vi "Controller Test Bench (2).vi"() -> ()   [LabVIEW 2022 SP3]
doc: "This example demonstrates how to continuously re-generate analog output data from a buffer in your computer's memory.\n\nRefer to your device documentation for pinouts and hardware capabilities."
uses:
  WhiteNoise.ctl
  <vilib>/Utility/error.llb/DialogType.ctl
  <vilib>/DAQmx/write.llb/DAQmx Write (Analog 1D Wfm NChan NSamp).vi
  <vilib>/DAQmx/read.llb/DAQmx Read (Analog Wfm 1Chan NSamp).vi
  <vilib>/DAQmx/create/channels.llb/DAQmx Create Channel (AO-Voltage-Basic).vi
  <vilib>/DAQmx/configure/timing.llb/DAQmx Timing (Sample Clock).vi
  <vilib>/measure/maspectr.llb/FFT Spectrum (Mag-Phase) for N Chan.vi
  <vilib>/DAQmx/miscellaneous.llb/DAQmx Fill In Error Info.vi
  <vilib>/DAQmx/create/channels.llb/DAQmx Create Channel (AI-Acceleration-Accelerometer).vi
  <vilib>/DAQmx/create/channels.llb/DAQmx Create Channel (AI-Force-IEPE Sensor).vi
  <vilib>/DAQmx/create/channels.llb/DAQmx Create Channel (AI-Sound Pressure-Microphone).vi
  <vilib>/measure/maspectr.llb/FFT Spectrum (Mag-Phase) for 1 Chan.vi
  <resource>/objmgr/daqmx.rc
  <vilib>/measure/NI_MABase.lvlib
  <vilib>/measure/NI_MAPro.lvlib
panel:
  in  "Start Output":bool
  out "Boolean 2":bool
  in  "Master Switch":bool
  in  "Start Control":bool
  in  "Start Input":bool
  in  "Tab Control":T1(tab)
  out "Actual Sample Rate":dbl=1000.0 format="%0.2f"
  in  "Physical Channel(s)":tag="Dev1/ao0"
  in  "Min Voltage":dbl=-3.0
  in  "Max Voltage":dbl=3.5
  in  "Sample Clock Source":tag="OnboardClock"
  in  "Sample Rate":dbl=40000.0
  in  "Stop":bool
  in  "Number of Samples":i32=40000
  out "Waveform Graph":waveform(dbl)[](graph)=[{"t0"=timestamp(0 s since 1904-01-01), "dt"=0.001, "Y"=[]}]
  out "Mag":cluster{"f0":dbl, "df":dbl, "magnitude":dbl[]}[](graph)
  out "Phase":cluster{"f0":dbl, "df":dbl, "phase":dbl[]}[](graph)
  in  "?":enum32{"White Noise", "Harmonic"}(tab)
  in  "Cluster":T3={"Seed"=0.0, "Standard Deviation"=0.2, "Reset"=FALSE, "Iterator"=1.0} {"Standard Deviation" format="%0.2p"}
  in  "Cluster 2":T4={"Iterator"=1.0, "Waveform Type"=0, "Frequency"=10.0, "Amplitude"=0.5} {"Amplitude" format="%0.2p"; "Frequency" format="%0.2p"; "Waveform Type" items=["Sine Wave", "Triangle Wave", "Square Wave", "Sawtooth Wave"]}
  in  "Task Type":T5(tab)
  in  "Min Acceleration":dbl=-100.0
  in  "Max Acceleration":dbl=100.0
  in  "Sensitivity [mV/g]":dbl=95.4
  in  "Physical Channel":tag="Dev1/ai0"
  in  "Sample Clock Source":tag="OnboardClock"
  in  "Sample Rate":dbl=40000.0
  in  "Terminal Configuration":i32(ring)=-1 items=["default"=-1, "RSE"=10083, "NRSE"=10078, "Differential"=10106, "Pseudodifferential"=12529]
  in  "Samples per Loop":i32=40000
  in  "Max Sound Pressure Level (dB)":dbl=120.0
  in  "Sound Pressure Units":i32(ring)=10081 items=["Pascals"=10081, "From Custom Scale"=10065]
  in  "Microphone Sensitivity":dbl=10.0
  in  "Sensitivity 2":dbl=50.0
  in  "Min Force":dbl=-100.0
  in  "Max Force":dbl=100.0
  in  "Sensitivity Units  2":i32(ring)=15891 items=["mVolts/N"=15891, "mVolts/lb"=15892]
  in  "Force Units":i32(ring)=15875 items=["Newtons"=15875, "Pounds"=15876, "From Custom Scale"=10065]
  in  "Window":dbl
  out "Boolean":bool
  in  "Restart Aaveraging":bool
  in  "Stop 2":bool
  out "Waveform Graph 2":waveform(dbl)(graph)
  out "Mag 2":cluster{"f0":dbl, "df":dbl, "magnitude":dbl[]}(graph)
  out "Phase 2":cluster{"f0":dbl, "df":dbl, "phase":dbl[]}(graph)
  in  "Reset Averaging":bool
  # "Channel Settings"
  # "Output"
  # "Timing and\nBuffer Settings"
  # "Waveform Settings"
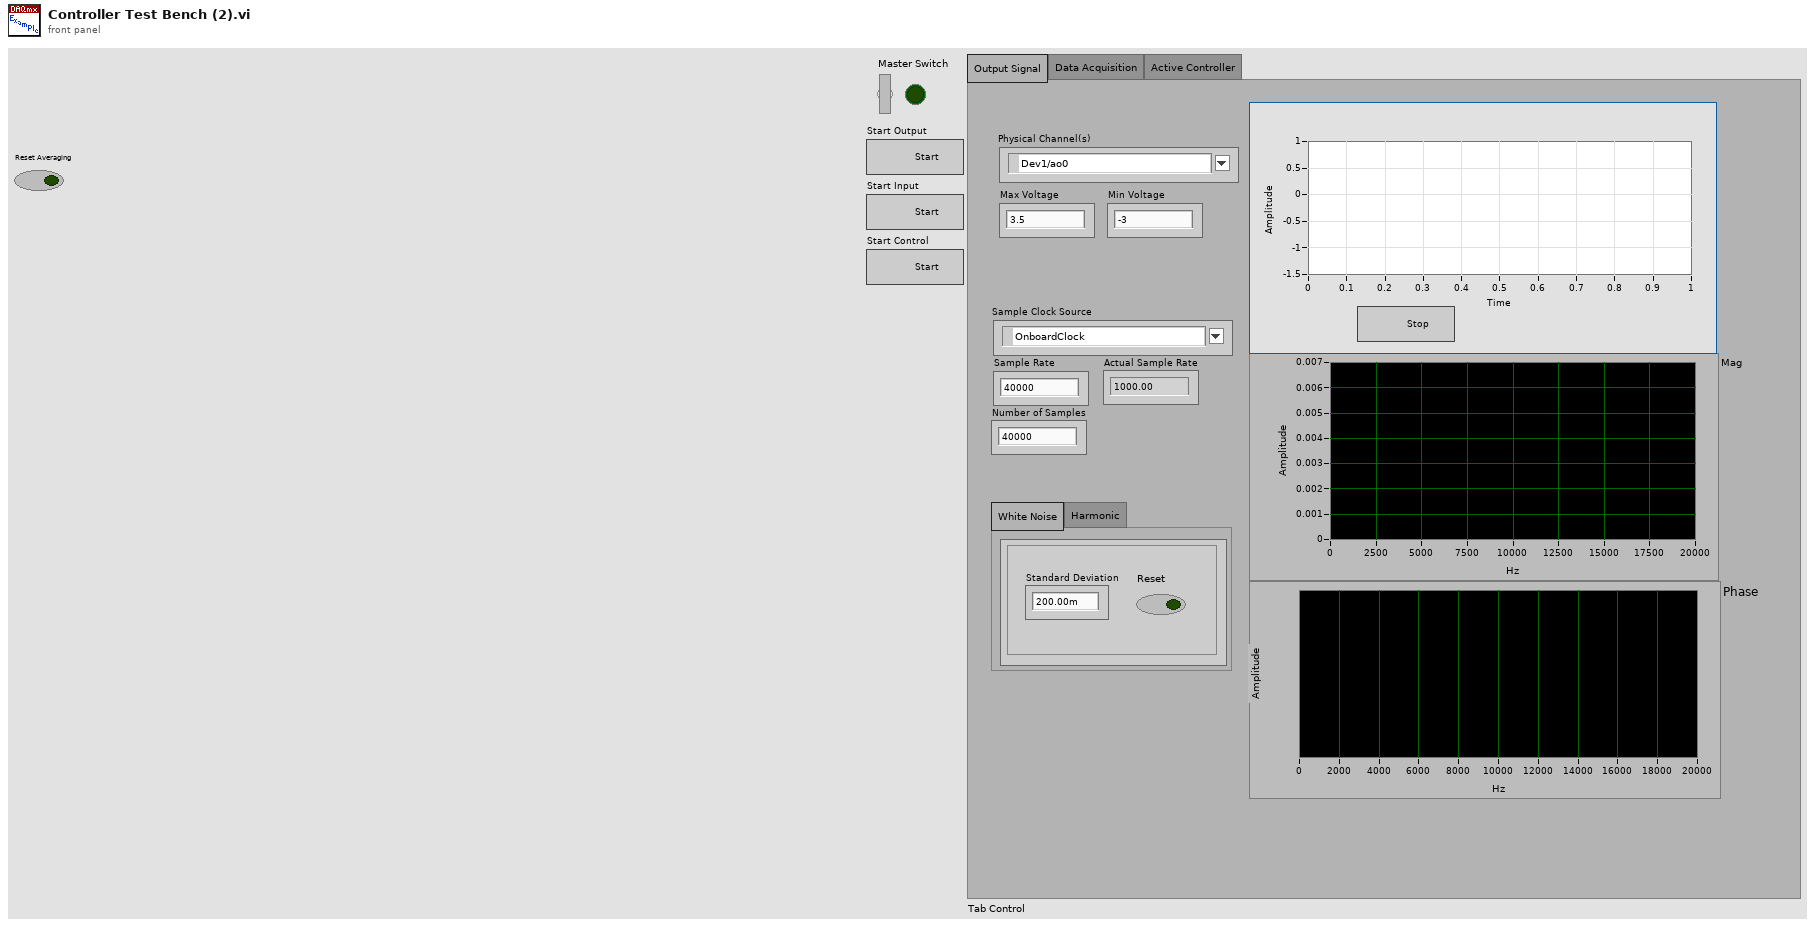
[diagram p1: front panel]
types:
  T1 = enum32{"Output Signal", "Data Acquisition", "Active Controller"}
  T2 = typedef "WhiteNoise.ctl" = dbl
  T3 = cluster{"Seed":T2, "Standard Deviation":dbl, "Reset":bool, "Iterator":dbl}
  T4 = cluster{"Iterator":dbl, "Waveform Type":u16, "Frequency":dbl, "Amplitude":dbl}
  T5 = enum32{"Acceleration", "Sound Pressure", "Force"}
  T6 = typedef "DialogType.ctl" = u16
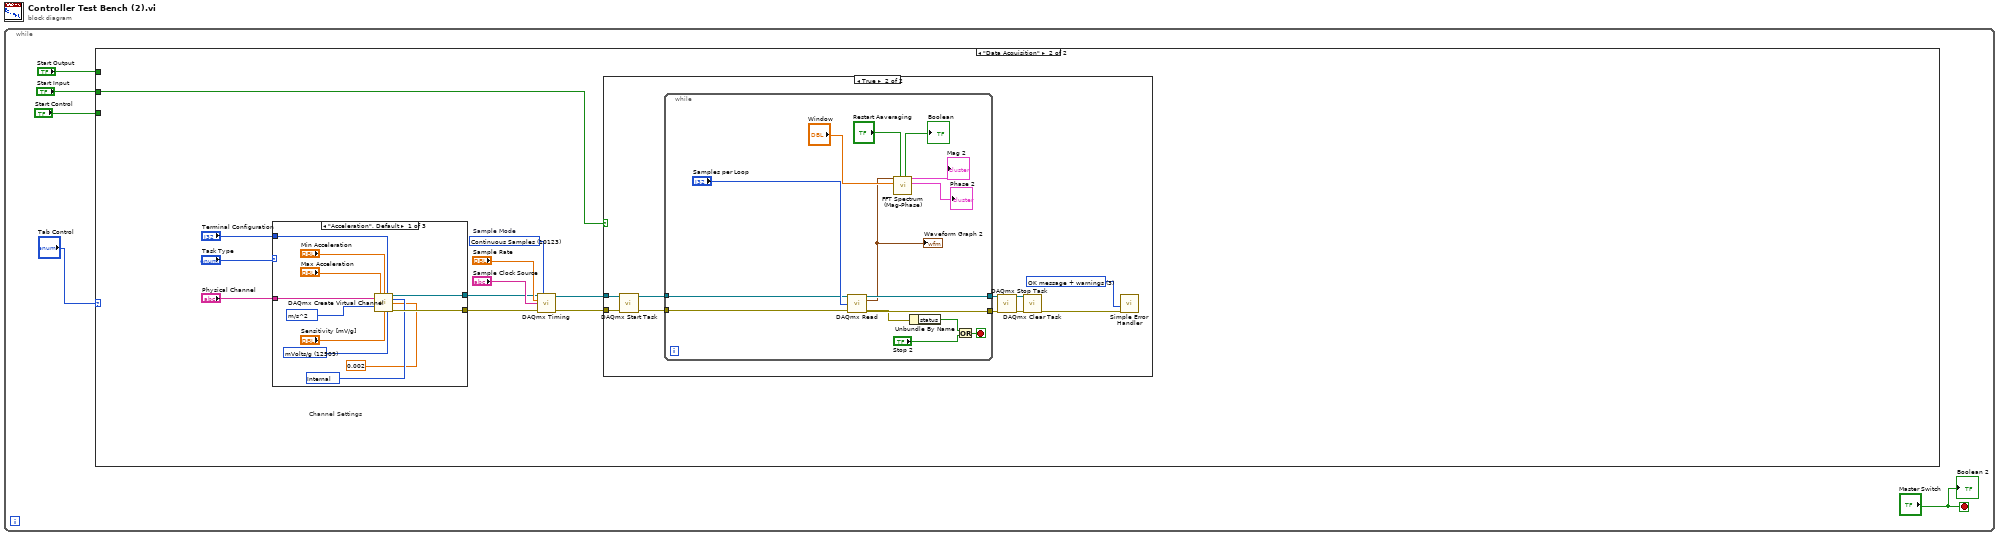
[diagram p0: block diagram]
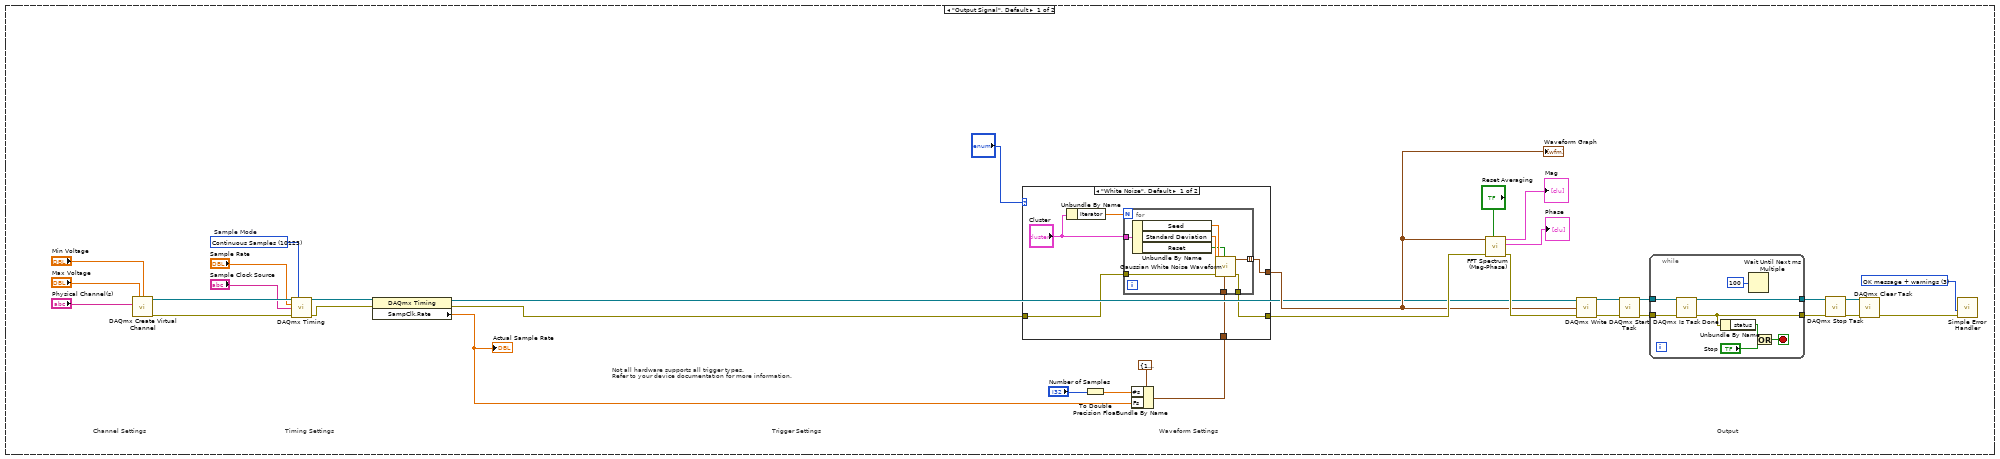
[diagram p2: hidden frame]
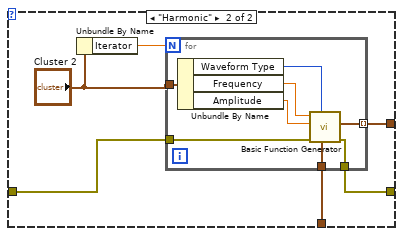
[diagram p3: hidden frame]
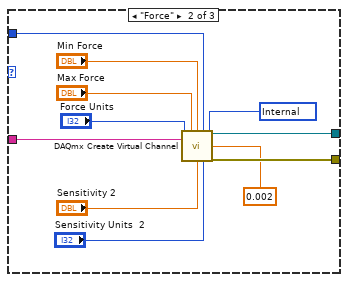
[diagram p5: hidden frame]
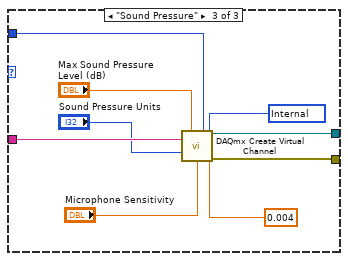
[diagram p6: hidden frame]
diagram:
  n1 = while {
    stop <- "Master Switch" stop-if-true
    n2 = case shown="\"Data Acquisition\"" "Tab Control" {
      tunnel: "Start Output" -> [_ _]
      tunnel: "Start Input" -> [_ w76]
      tunnel: "Start Control" -> [_ _]
      frame "Output Signal", Default {
        w16 = T6 3 items=["no dialog", "OK message", "continue or stop message", "OK message + warnings", "continue/stop + warnings"] ("type of dialog (OK msg:1)")
        w37 = 10123 items=["Finite Samples"=10178, "Continuous Samples"=10123, "Hardware Timed Single Point"=12522]  # Sample Mode
        # "Trigger Settings"
        # "Not all hardware supports all trigger types.\nRefer to your device documentation for more information."
        # "Output"
        # "Waveform Settings"
        # "Timing Settings"
        # "Channel Settings"
        n3 = call-poly <vilib>:"DAQmx Create Virtual Channel.vi"("maximum value"="Max Voltage", "minimum value"="Min Voltage", "physical channels"="Physical Channel(s)") -> ("task out"=w35:refnum<k21>, "error out"=w36:errorcluster)  [unwired: 11 in]
        n4 = call-poly <vilib>:"DAQmx Timing.vi"("task/channels in"=w35, "sample mode"=w37, "rate"="Sample Rate", "source"="Sample Clock Source", "error in"=w36) -> ("task out"=w39:refnum<k21>, "error out"=w38:errorcluster)  [unwired: 9 in]
        n5 = property class="DAQmx Timing"(reference=w39, error in=w38) -> (reference out=w7:refnum<k21>, error out=w6:errorcluster, "SampClk.Rate"=w25:dbl)
        "Actual Sample Rate" <- w25
        n6 = To Double Precision Float(number="Number of Samples") -> (double precision float=w22:dbl)
        n7 = Bundle By Name(cluster=cluster{"Fs":dbl, "#s":dbl} {"Fs"=1000.0, "#s"=1000.0} ("sampling info"), "#s"=w22, "Fs"=w25) -> (w24:cluster{"Fs":dbl, "#s":dbl})
        n8 = case shown="\"White Noise\", Default" "?" {
          tunnel: w24 -> [w45 w57]
          tunnel: w6 -> [w44 w59]
          tunnel: [w43 w56] -> w10
          tunnel: [w40 w58] -> w9
          frame "White Noise", Default {
            n9 = Unbundle By Name("Cluster") -> ("Iterator"=w42:dbl)
            n10 = for {
              N: w42 -> [_]
              tunnel: w44 -> [w53]
              tunnel: w45 -> [w52]
              tunnel: [w51] -> w43
              tunnel: "Cluster" -> [w50]
              tunnel: [w49] -> w40 mode=indexing
              n11 = Unbundle By Name(w50) -> ("Seed"=w48:T2, "Standard Deviation"=w47:dbl, "Reset"=w46:bool)
              n12 = call <vilib>:"Gaussian White Noise Waveform.vi"("sampling info"=w52, "reset signal"=w46, "error in (no error)"=w53, "seed"=w48, "standard deviation"=w47) -> ("error out"=w51:errorcluster, "signal out"=w49:waveform(dbl))  [unwired: 5 in]
            }
          }
          frame "Harmonic" {
            n13 = Unbundle By Name("Cluster 2") -> ("Iterator"=w55:dbl)
            n14 = for {
              N: w55 -> [_]
              tunnel: w59 -> [w67]
              tunnel: w57 -> [w66]
              tunnel: [w65] -> w56
              tunnel: "Cluster 2" -> [w64]
              tunnel: [w60] -> w58 mode=indexing
              n15 = Unbundle By Name(w64) -> ("Waveform Type"=w63:u16, "Frequency"=w62:dbl, "Amplitude"=w61:dbl)
              n16 = call <vilib>:"Basic Function Generator.vi"("sampling info"=w66, "signal type"=w63, "error in (no error)"=w67, "amplitude"=w61, "frequency"=w62) -> ("error out"=w65:errorcluster, "signal out"=w60:waveform(dbl))  [unwired: 4 in, 1 out]
            }
          }
        }
        "Waveform Graph" <- w9
        n17 = call-poly <vilib>:"FFT Spectrum (Mag-Phase).vi"("restart averaging (F)"="Reset Averaging", "error in (no error)"=w10, "time signals"=w9) -> ("error out"=w11:errorcluster, "phases"=→"Phase":cluster{"f0":dbl, "df":dbl, "phase":dbl[]}[], "magnitudes"=→"Mag":cluster{"f0":dbl, "df":dbl, "magnitude":dbl[]}[])  [unwired: 4 in, 2 out]
        n18 = call-poly <vilib>:"DAQmx Write.vi"("task/channels in"=w7, "data"=w9, "error in"=w11) -> ("task out"=w23:refnum<k21>, "error out"=w15:errorcluster)  [unwired: 10 in, 1 out]
        n19 = call <vilib>:"DAQmx Start Task.vi"("task/channels in"=w23, "error in"=w15) -> ("task out"=w34:refnum<k21>, "error out"=w33:errorcluster)  [unwired: 12 in]
        n20 = while {
          tunnel: w34 -> [w75]
          tunnel: w33 -> [w74]
          tunnel: [w71] -> w17
          tunnel: [w72] -> w18
          stop <- w73 stop-if-true
          n21 = call <vilib>:"DAQmx Is Task Done.vi"("task/channels in"=w75, "error in"=w74) -> ("task out"=w72:refnum<k21>, "error out"=w71:errorcluster)  [unwired: 11 in, 1 out]
          n22 = Unbundle By Name(w71) -> ("status"=w70:bool)
          n23 = Wait Until Next ms Multiple(millisecond multiple=u32 100) -> ()  [unwired: 1 out]
          n24 = Or(x=w70, y="Stop") -> (x .or. y?=w73:bool)
        }
        n25 = call <vilib>:"DAQmx Stop Task.vi"("task/channels in"=w18, "error in"=w17) -> ("task out"=w20:refnum<k21>, "error out"=w19:errorcluster)  [unwired: 12 in]
        n26 = call <vilib>:"DAQmx Clear Task.vi"("task in"=w20, "error in"=w19) -> ("error out"=w32:errorcluster)  [unwired: 13 in]
        n27 = call <vilib>:"Simple Error Handler.vi"("type of dialog (OK msg:1)"=w16, "error in (no error)"=w32) -> ()  [unwired: 3 in, 5 out]
      }
      frame "Data Acquisition" {
        w86 = 10123 items=["Finite Samples"=10178, "Continuous Samples"=10123, "Hardware Timed Single Point"=12522]  # Sample Mode
        # "Channel Settings"
        n28 = case shown="\"Acceleration\", Default" "Task Type" {
          tunnel: [w113 w124 w135] -> w77
          tunnel: [w121 w132 w141] -> w80
          tunnel: "Physical Channel" -> [w120 w131 w140]
          tunnel: "Terminal Configuration" -> [w119 w130 w139]
          frame "Acceleration", Default {
            w112 = 10200 items=["Internal"=10200, "External"=10167, "None"=10230] ("IEPE Excitation Source")
            w115 = 12470 items=["g"=10186, "m/s^2"=12470, "in/s^2"=12471, "From Custom Scale"=10065] ("Acceleration Units")
            w114 = 12509 items=["mVolts/ms^2"=0, "mVolts/g"=12509, "Volts/g"=12510] ("Sensitivity Units")
            n29 = call-poly <vilib>:"DAQmx Create Virtual Channel.vi"("maximum value"="Max Acceleration", "minimum value"="Min Acceleration", "input terminal configuration"=w119, "physical channels"=w120, "current excitation source"=w112, "current excitation value"=0.002 ("IEPE Current Value (A)"), "units"=w115, "sensitivity"="Sensitivity [mV/g]", "sensitivity units"=w114) -> ("task out"=w121:refnum<k21>, "error out"=w113:errorcluster)  [unwired: 5 in]
          }
          frame "Force" {
            w122 = 10200 items=["Internal"=10200, "External"=10167, "None"=10230] ("current excitation source")
            n30 = call-poly <vilib>:"DAQmx Create Virtual Channel.vi"("maximum value"="Max Force", "minimum value"="Min Force", "input terminal configuration"=w130, "physical channels"=w131, "current excitation source"=w122, "current excitation value"=0.002, "units"="Force Units", "sensitivity"="Sensitivity 2", "sensitivity units"="Sensitivity Units  2") -> ("task out"=w132:refnum<k21>, "error out"=w124:errorcluster)  [unwired: 5 in]
          }
          frame "Sound Pressure" {
            w133 = 10200 items=["Internal"=10200, "External"=10167, "None"=10230] ("current excitation source")
            n31 = call-poly <vilib>:"DAQmx Create Virtual Channel.vi"("maximum sound pressure level"="Max Sound Pressure Level (dB)", "input terminal configuration"=w139, "physical channels"=w140, "current excitation source"=w133, "current excitation value"=0.004, "units"="Sound Pressure Units", "microphone sensitivity"="Microphone Sensitivity") -> ("task out"=w141:refnum<k21>, "error out"=w135:errorcluster)  [unwired: 7 in]
          }
        }
        n32 = call-poly <vilib>:"DAQmx Timing.vi"("task/channels in"=w80, "sample mode"=w86, "rate"="Sample Rate", "source"="Sample Clock Source", "error in"=w77) -> ("task out"=w78:refnum<k21>, "error out"=w79:errorcluster)  [unwired: 9 in]
        n33 = case shown="True" w76 {
          tunnel: w79 -> [_ w88]
          tunnel: w78 -> [_ w87]
          frame False {
          }
          frame True {
            w94 = T6 3 items=["no dialog", "OK message", "continue or stop message", "OK message + warnings", "continue/stop + warnings"] ("type of dialog (OK msg:1)")
            n34 = call <vilib>:"DAQmx Start Task.vi"("task/channels in"=w87, "error in"=w88) -> ("task out"=w92:refnum<k21>, "error out"=w91:errorcluster)  [unwired: 12 in]
            n35 = while {
              tunnel: w92 -> [w98]
              tunnel: w91 -> [w97]
              tunnel: [w108] -> w90
              tunnel: [w101] -> w89
              stop <- w100 stop-if-true
              n36 = call-poly <vilib>:"DAQmx Read.vi"("task/channels in"=w98, "number of samples per channel"="Samples per Loop", "error in"=w97) -> ("task out"=w108:refnum<k21>, "data"=w99:waveform(dbl), "error out"=w101:errorcluster)  [unwired: 10 in]
              "Waveform Graph 2" <- w99
              n37 = call-poly <vilib>:"FFT Spectrum (Mag-Phase).vi"("restart averaging (F)"="Restart Aaveraging", "window"="Window", "time signal"=w99) -> ("phase"=→"Phase 2":cluster{"f0":dbl, "df":dbl, "phase":dbl[]}, "magnitude"=→"Mag 2":cluster{"f0":dbl, "df":dbl, "magnitude":dbl[]}, "averaging done"=→"Boolean":bool)  [unwired: 4 in, 2 out]
              n38 = Unbundle By Name(w97) -> ("status"=w110:bool)
              n39 = Or(x=w110, y="Stop 2") -> (x .or. y?=w100:bool)
            }
            n40 = call <vilib>:"DAQmx Stop Task.vi"("task/channels in"=w90, "error in"=w89) -> ("task out"=w96:refnum<k21>, "error out"=w95:errorcluster)  [unwired: 12 in]
            n41 = call <vilib>:"DAQmx Clear Task.vi"("task in"=w96, "error in"=w95) -> ("error out"=w93:errorcluster)  [unwired: 13 in]
            n42 = call <vilib>:"Simple Error Handler.vi"("type of dialog (OK msg:1)"=w94, "error in (no error)"=w93) -> ()  [unwired: 3 in, 5 out]
          }
        }
      }
    }
    "Boolean 2" <- "Master Switch"
  }
